vi "zernike_from_xy.vi"(1 "y (-.5 to .5)":dbl, 2 "x (-.5 to .5)":dbl, 3 "Numeric":i32) -> (0 "z":dbl)   [LabVIEW 2019]
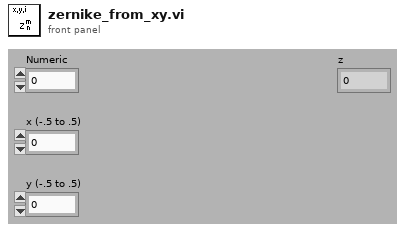
[diagram p1: front panel]
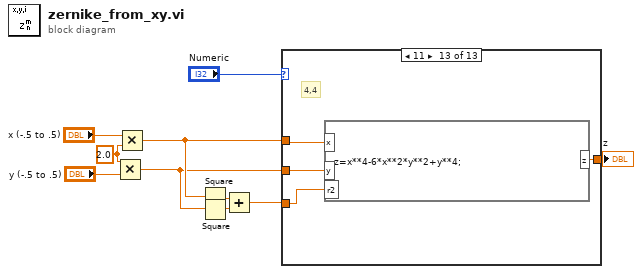
[diagram p0: block diagram]
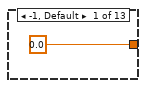
[diagram p2: hidden frame]
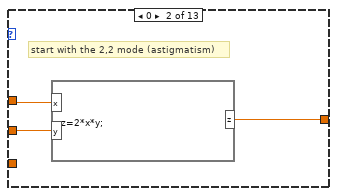
[diagram p3: hidden frame]
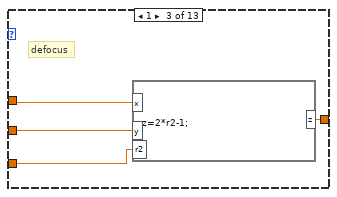
[diagram p4: hidden frame]
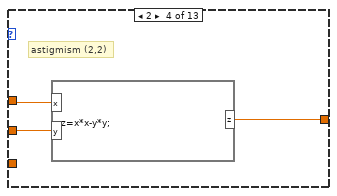
[diagram p5: hidden frame]
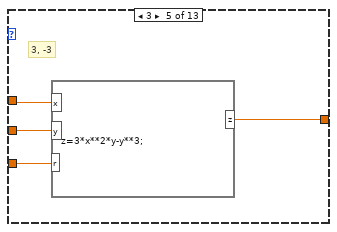
[diagram p6: hidden frame]
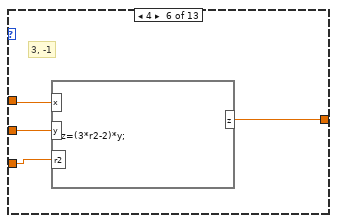
[diagram p7: hidden frame]
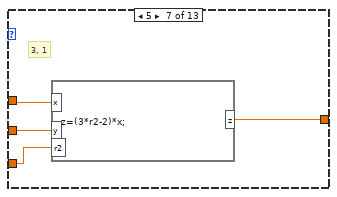
[diagram p8: hidden frame]
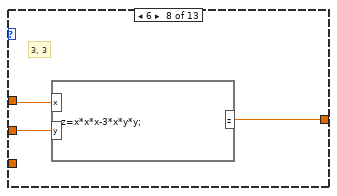
[diagram p9: hidden frame]
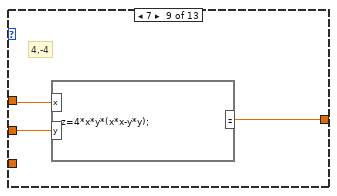
[diagram p10: hidden frame]
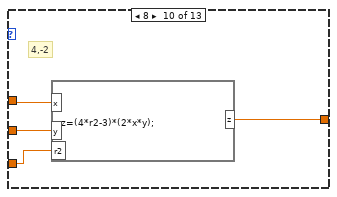
[diagram p11: hidden frame]
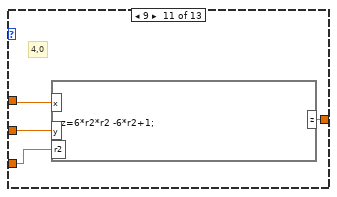
[diagram p12: hidden frame]
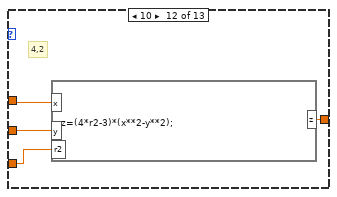
[diagram p13: hidden frame]
diagram:
  w2 = 2.0 ("x")
  n1 = Multiply(x=w2, y="y (-.5 to .5)") -> (x*y=w3:dbl)
  n2 = Multiply(x="x (-.5 to .5)", y=w2) -> (x*y=w4:dbl)
  n3 = Square(x=w4) -> (x^2=w7:dbl)
  n4 = Square(x=w3) -> (x^2=w8:dbl)
  n5 = Add(x=w7, y=w8) -> (x+y=w1:dbl)
  n6 = case shown="11" "Numeric" {
    tunnel: w4 -> [_ w14 w16 w21 w25 w29 w33 w36 w39 w43 w47 w51 w55]
    tunnel: w3 -> [_ w13 w17 w20 w24 w28 w32 w35 w38 w42 w46 w50 w54]
    tunnel: [0.0 ("z") w12 w18 w19 w23 w27 w31 w34 w37 w41 w45 w49 w53] -> w9
    tunnel: w1 -> [_ _ w15 _ w22 w26 w30 _ _ w40 w44 w48 w52]
    frame -1, Default {
    }
    frame 0 {
      # "start with the 2,2 mode (astigmatism)"
      n7 = formula code="z=2*x*y;"("x"=w14, "y"=w13) -> ("z"=w12:dbl)
    }
    frame 1 {
      # "defocus"
      n8 = formula code="z=2*r2-1;"("x"=w16, "y"=w17, "r2"=w15) -> ("z"=w18:dbl)
    }
    frame 2 {
      # "astigmism (2,2)"
      n9 = formula code="z=x*x-y*y;"("x"=w21, "y"=w20) -> ("z"=w19:dbl)
    }
    frame 3 {
      # "3, -3"
      n10 = formula code="z=3*x**2*y-y**3;"("x"=w25, "y"=w24, "r"=w22) -> ("z"=w23:dbl)
    }
    frame 4 {
      # "3, -1"
      n11 = formula code="z=(3*r2-2)*y;"("x"=w29, "y"=w28, "r2"=w26) -> ("z"=w27:dbl)
    }
    frame 5 {
      # "3, 1"
      n12 = formula code="z=(3*r2-2)*x;"("x"=w33, "y"=w32, "r2"=w30) -> ("z"=w31:dbl)
    }
    frame 6 {
      # "3, 3"
      n13 = formula code="z=x*x*x-3*x*y*y;"("x"=w36, "y"=w35) -> ("z"=w34:dbl)
    }
    frame 7 {
      # "4,-4"
      n14 = formula code="z=4*x*y*(x*x-y*y);"("x"=w39, "y"=w38) -> ("z"=w37:dbl)
    }
    frame 8 {
      # "4,-2"
      n15 = formula code="z=(4*r2-3)*(2*x*y);"("x"=w43, "y"=w42, "r2"=w40) -> ("z"=w41:dbl)
    }
    frame 9 {
      # "4,0"
      n16 = formula code="z=6*r2*r2 -6*r2+1;"("x"=w47, "y"=w46, "r2"=w44) -> ("z"=w45:dbl)
    }
    frame 10 {
      # "4,2"
      n17 = formula code="z=(4*r2-3)*(x**2-y**2);"("x"=w51, "y"=w50, "r2"=w48) -> ("z"=w49:dbl)
    }
    frame 11 {
      # "4,4"
      n18 = formula code="z=x**4-6*x**2*y**2+y**4;"("x"=w55, "y"=w54, "r2"=w52) -> ("z"=w53:dbl)
    }
  }
  "z" <- w9
